vi "LoggingExample.vi"() -> ()   [LabVIEW 2015]
uses:
  Packet Types.ctl
panel:
  in  "File Name":string="log1.csv"
  in  "Header String":string="value 1, value 2, value 3"
  out "Line Written":bool=TRUE
  in  "Value 3":string="hey hey"
  in  "stop":bool
  in  "Logging Frequency":dbl(slide)=1.022434770467647 scale=0.1..20.0
  in  "Value 2":dbl(slide)=4.8979591836734695 scale=0.0..10.0
  in  "Value 1":dbl(slide)=2.3469387755102042 scale=0.0..10.0
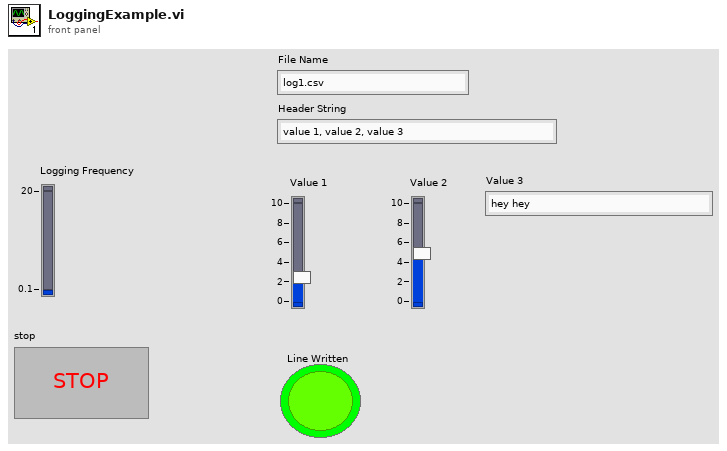
[diagram p1: front panel]
types:
  T1 = typedef "Packet Types.ctl" = enum16{"Log line", "Open File", "Send Header", "Set Time", "Send to LCD", "Close File"}
  T2 = typedef "WPI_SerialPortRef.ctl" = cluster{"DevStatus":errorcluster, "Serial Port Name":refnum<visa-resource-name>}
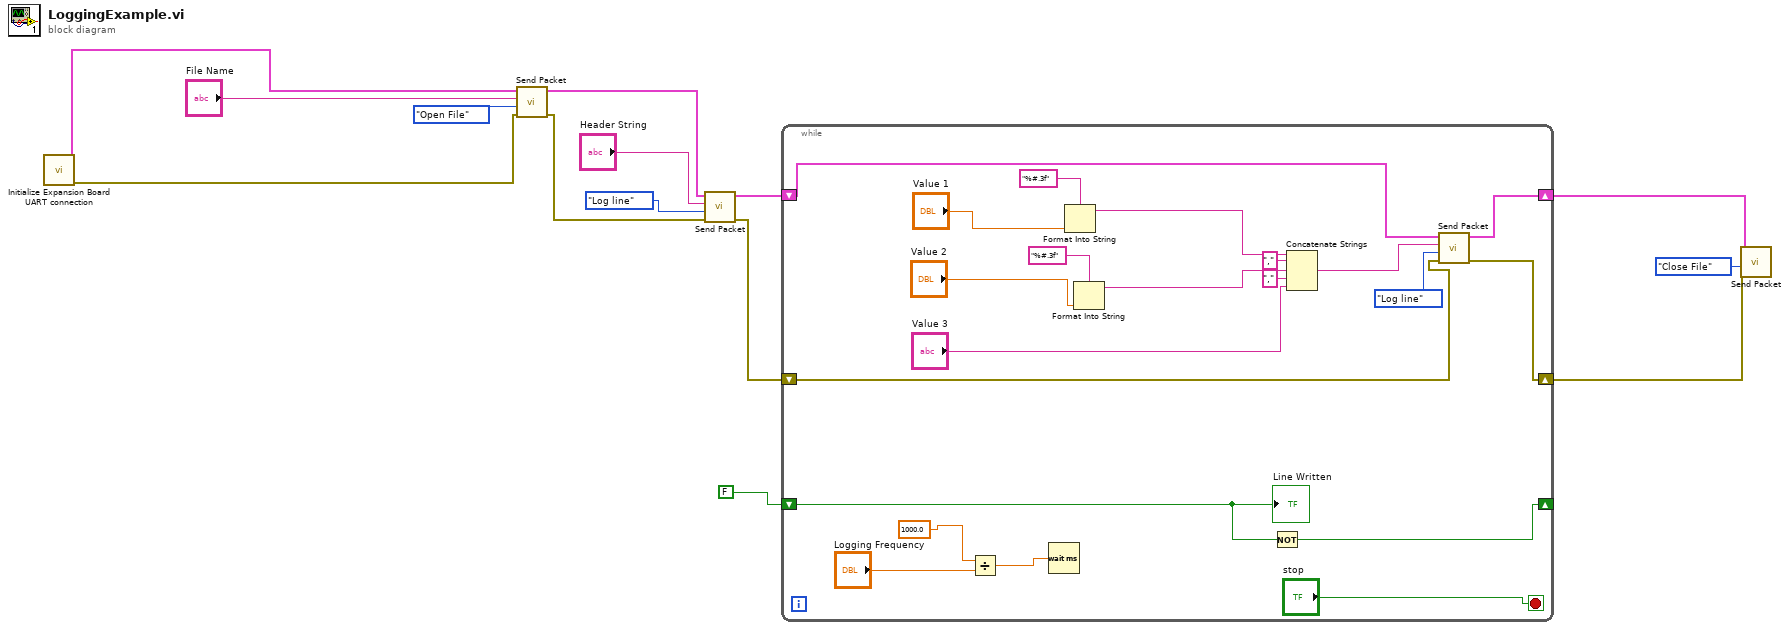
[diagram p0: block diagram]
diagram:
  n1 = call "Initialize Expansion Board UART connection.vi"() -> ("error out"=w11:errorcluster, "SerialPortRef"=w13:T2)  [unwired: 10 in]
  n2 = call "Send Packet.vi"("error in (no error) 2"=w11, 7:Packet_Types."Open File", "Log string 2"="File Name", "SerialPortRef 2"=w13) -> ("error out 2"=w10:errorcluster, "SerialPortRef out 2"=w7:T2)  [unwired: 4 in]
  n3 = call "Send Packet.vi"("error in (no error) 2"=w10, 7:Packet_Types."Log line", "Log string 2"="Header String", "SerialPortRef 2"=w7) -> ("error out 2"=w5:errorcluster, "SerialPortRef out 2"=w6:T2)  [unwired: 4 in]
  n4 = while {
    shift-right: [w24] -> _
    shift-left: FALSE -> [w25]
    shift-right: [w15] -> w4
    shift-left: w6 -> [w17]
    shift-right: [w16] -> w3
    shift-left: w5 -> [w20]
    stop <- "stop" stop-if-true
    n5 = Divide(x=1000.0, y="Logging Frequency") -> (x/y=w23:dbl)
    n6 = Wait (ms)(milliseconds to wait=w23) -> ()  [unwired: 1 out]
    n7 = Format Into String(format string="%#.3f", "Value 1") -> (resulting string=w30:string)  [unwired: 2 in, 1 out]
    n8 = Format Into String(format string="%#.3f", "Value 2") -> (resulting string=w31:string)  [unwired: 2 in, 1 out]
    n9 = Not(x=w25) -> (.not. x?=w24:bool)
    n10 = Concatenate Strings(w30, "," ("string"), w31, "," ("string"), "Value 3") -> (w18:string)
    n11 = call "Send Packet.vi"("error in (no error) 2"=w20, 7:Packet_Types."Log line", "Log string 2"=w18, "SerialPortRef 2"=w17) -> ("error out 2"=w16:errorcluster, "SerialPortRef out 2"=w15:T2)  [unwired: 4 in]
    "Line Written" <- w25
  }
  n12 = call "Send Packet.vi"("error in (no error) 2"=w3, 7:Packet_Types."Close File", "SerialPortRef 2"=w4) -> ()  [unwired: 5 in, 2 out]
